vi "Configure Trigger (Pattern).vi"(0 "VISA resource name":refnum<visa-resource-name>, 1 "B Pattern Code (0: H)":i32(ring) items=["H", "L", "X", "R", "F"], 2 "Trigger Level (0)":dbl, 3 "Qualifier (0: None)":i32(ring) items=["None", "Greater", "Less", "InRange", "OutRange"], 5 "A Pattern Code (0: H)":i32(ring) items=["H", "L", "X", "R", "F"], 7 "Signal Source A (0: Channel 1)":i32(ring) items=["Channel 1", "Channel 2", "Channel 3", "Channel 4"], 9 "Signal Source B (0: Channel 1)":i32(ring)=1 items=["Channel 1", "Channel 2", "Channel 3", "Channel 4"], 11 "error in (no error)":errorcluster, 12 "Upper Limit (2E-6 s)":dbl=2e-06, 13 "Lower Limit (1E-6 s)":dbl=1e-06) -> (4 "VISA resource name out":refnum<visa-resource-name>, 15 "error out":errorcluster)   [LabVIEW 2015, in "ZhiYuan ZDS Series for TCP.lvlib"]
doc: "Configures the setting for pattern trigger."
uses:
  ZhiYuan ZDS Series for TCP.lvlib
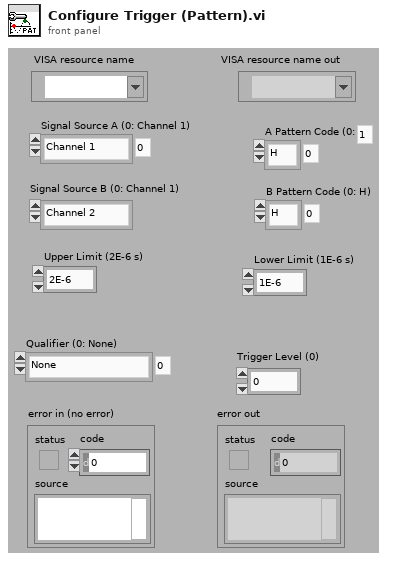
[diagram p1: front panel]
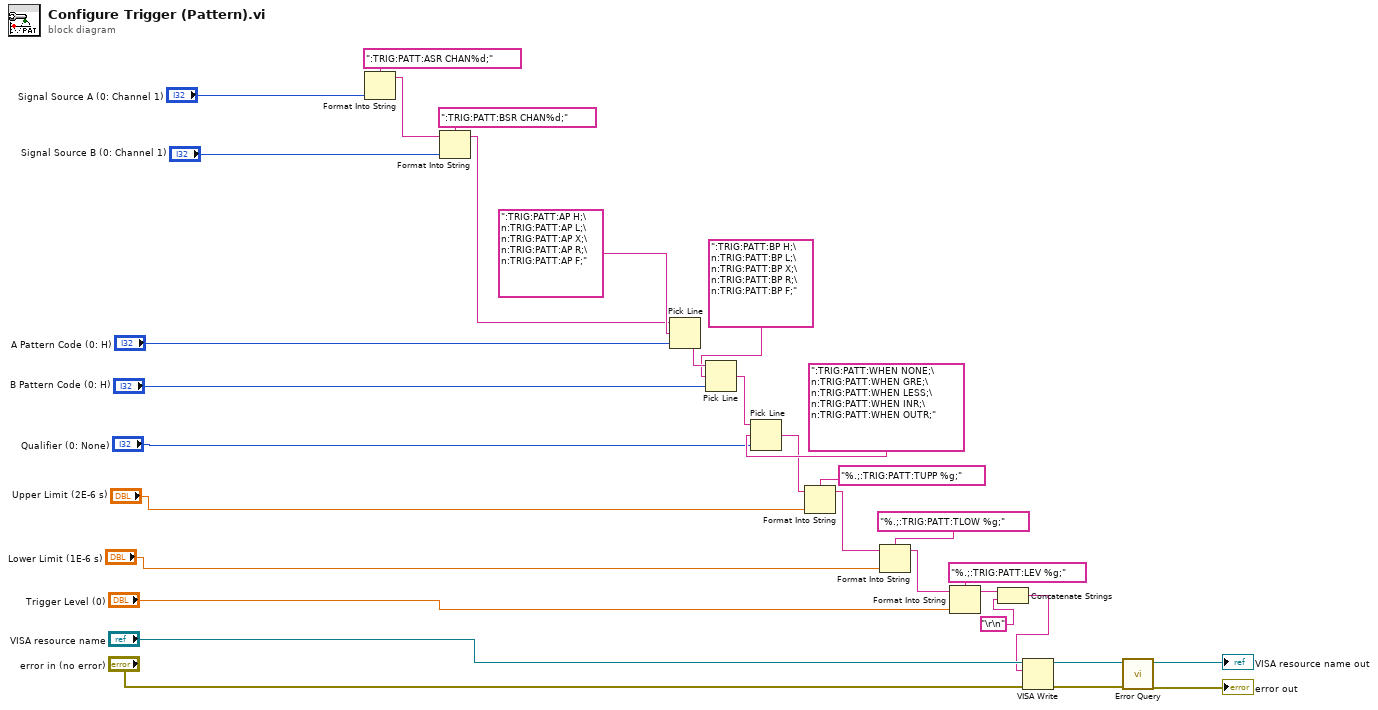
[diagram p0: block diagram]
diagram:
  n1 = Format Into String(format string=":TRIG:PATT:ASR CHAN%d;", "Signal Source A (0: Channel 1)") -> (resulting string=w19:string)  [unwired: 2 in, 1 out]
  n2 = Format Into String(format string=":TRIG:PATT:BSR CHAN%d;", initial string=w19, "Signal Source B (0: Channel 1)") -> (resulting string=w15:string)  [unwired: 1 in, 1 out]
  n3 = Pick Line(string ("")=w15, multi-line string=":TRIG:PATT:AP H;\n:TRIG:PATT:AP L;\n:TRIG:PATT:AP X;\n:TRIG:PATT:AP R;\n:TRIG:PATT:AP F;", line index="A Pattern Code (0: H)") -> (output string=w23:string)
  n4 = Pick Line(string ("")=w23, multi-line string=":TRIG:PATT:BP H;\n:TRIG:PATT:BP L;\n:TRIG:PATT:BP X;\n:TRIG:PATT:BP R;\n:TRIG:PATT:BP F;", line index="B Pattern Code (0: H)") -> (output string=w13:string)
  n5 = Pick Line(string ("")=w13, multi-line string=":TRIG:PATT:WHEN NONE;\n:TRIG:PATT:WHEN GRE;\n:TRIG:PATT:WHEN LESS;\n:TRIG:PATT:WHEN INR;\n:TRIG:PATT:WHEN OUTR;", line index="Qualifier (0: None)") -> (output string=w9:string)
  n6 = Format Into String(format string="%.;:TRIG:PATT:TUPP %g;", initial string=w9, "Upper Limit (2E-6 s)") -> (resulting string=w8:string)  [unwired: 1 in, 1 out]
  n7 = Format Into String(format string="%.;:TRIG:PATT:TLOW %g;", initial string=w8, "Lower Limit (1E-6 s)") -> (resulting string=w4:string)  [unwired: 1 in, 1 out]
  n8 = Format Into String(format string="%.;:TRIG:PATT:LEV %g;", initial string=w4, "Trigger Level (0)") -> (resulting string=w3:string)  [unwired: 1 in, 1 out]
  n9 = Concatenate Strings(w3, "\r\n") -> (w1:string)
  n10 = VISA Write(VISA resource name="VISA resource name", write buffer=w1, error in (no error)="error in (no error)") -> (VISA resource name out=w27:refnum<visa-resource-name>, error out=w26:errorcluster)  [unwired: 1 out]
  n11 = call "Error Query.vi"("error in (no error)"=w26, "VISA resource name"=w27) -> ("error out"=→"error out":errorcluster, "VISA resource name out"=→"VISA resource name out":refnum<visa-resource-name>)  [unwired: 6 in, 2 out]
